vi "Read Data.vi"() -> ()   [LabVIEW 2010]
doc: "이 VI는 LabVIEW Core II 과정의 글로벌 데이터 프로젝트 연습문제에 대한 해답입니다.\n\n이 프로젝트를 실행하려면 글로벌 데이터 LV 프로젝트 파일을 열고, 데이터 생성 VI 및 데이터 읽기 VI를 열고 이 두 VI를 실행하십시오. 데이터 생성 VI에서 데이터를 생성하고 데이터 읽기 VI에서 디스플레이합니다. 두 개 VI는 단일 정지 버튼을 공유하고 있습니다."
panel:
  in  "정지":bool
  out "데이터 차트":dbl(graph)
  in  "시간 지연 (ms)":u32(slide) scale=0.0..200.0
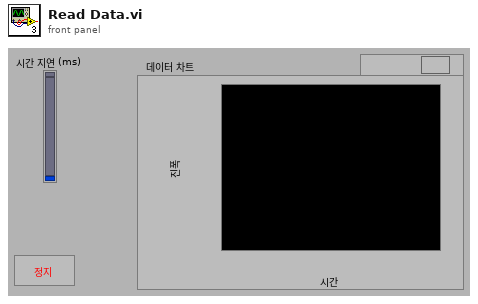
[diagram p1: front panel]
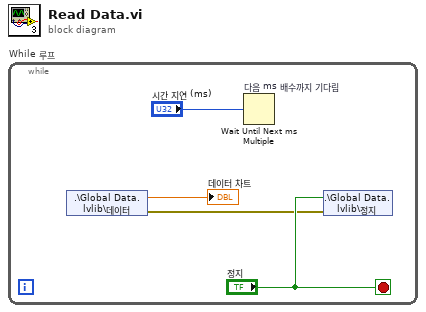
[diagram p0: block diagram]
diagram:
  n1 = while "While 루프" {
    stop <- "정지" stop-if-true
    n2 = shared-variable ".\\Global Data.lvlib\\데이터"() -> (→"데이터 차트":dbl, error out=w1:errorcluster)  [unwired: 1 in]
    n3 = Wait Until Next ms Multiple "다음 ms 배수까지 기다림"(millisecond multiple="시간 지연 (ms)") -> ()  [unwired: 1 out]
    n4 = shared-variable ".\\Global Data.lvlib\\정지"("정지", error in=w1) -> ()  [unwired: 1 out]
  }
